vi "Analyze Coefficients-Quantized Multirate Filter.vi"() -> ()   [LabVIEW 2023]
doc: "Demonstrates how to use the DFD FXP MRate Quantization VI to quantize the coefficients of a floating-point multirate filter and use the DFD Plot MRate Freq Response VI to analyze a quantized multirate filter.\n\n1) Complete the following steps to use this VI.Run the VI. This VI designs a floating-point multirate filter with the specifications in the <B>Design Settings</B> section. This VI then quantize the multirate filter coefficients.\n2) Observe the Magnitude Responses graph. This graph displays the magnitude responses of both the fixed-point multirate filter and the reference floating-point multirate filter. You also can observe the Phase Responses graph for more information.\n3) Modify the <B>Quantization Settings</B> and run this VI again. Observe the Magnitude Responses graph to see how your changes affect the magnitude response of the fixed-point multirate filter.\n4) Examine the block diagram of this VI to obtain information about using the DFD FXP MRate Quantization Vi and the DFD Plot MRate Freq Response VI."
uses:
  <vilib>/addons/Digital Filter Design/_Objects.llb/DFD Multirate Filter Specification (Design).ctl
  <vilib>/addons/Digital Filter Design/_Objects.llb/DFD Filter Ripple Specification (Design).ctl
  <vilib>/addons/Digital Filter Design/_Objects.llb/DFD Coef Norm Type.ctl
  <vilib>/addons/Digital Filter Design/_Objects.llb/DFD Multirate Filtering Mode.ctl
  <vilib>/addons/Digital Filter Design/_Objects.llb/DFD Phase Setting.ctl
  <vilib>/addons/Digital Filter Design/Design.llb/DFD MRate Filter Design (Integer).vi
  <vilib>/addons/Digital Filter Design/NI_DigFilterLicensed.lvlib
panel:
  in  "dB on?":bool=TRUE
  in  "Phase View":T1
  out "Phase Responses":cluster{"f0":dbl, "df":dbl, "values":dbl[]}[](graph)
  out "Error Message":string
  out "Magnitude Responses":cluster{"f0":dbl, "df":dbl, "values":dbl[]}[](graph)
  in  "Filtering Mode":T2=2 items=["No Rate Change", "Interpolation", "Decimation"]
  in  "Factor":i32=8
  in  "Coefficients Word Length":i16=16
  in  "Scale by Power of 2?":bool
  in  "Scale Type":T3=enum."Time Domain 1-Norm"
  in  "Ripple Specifications":T4={"passband"=0.1, "stopband"=60.0, "dB/linear? (T: dB)"=TRUE}
  in  "Input Sampling Frequency [Hz]":dbl=800.0
  in  "Frequency Specifications [Hz]":T5={"fpass"=45.0, "fstop"=52.0}
  # "Select Help>>Show Context Help and move the cursor over the VI icon for more information."
  # "Design Settings"
  # "Quantization Settings"
  # "View Settings"
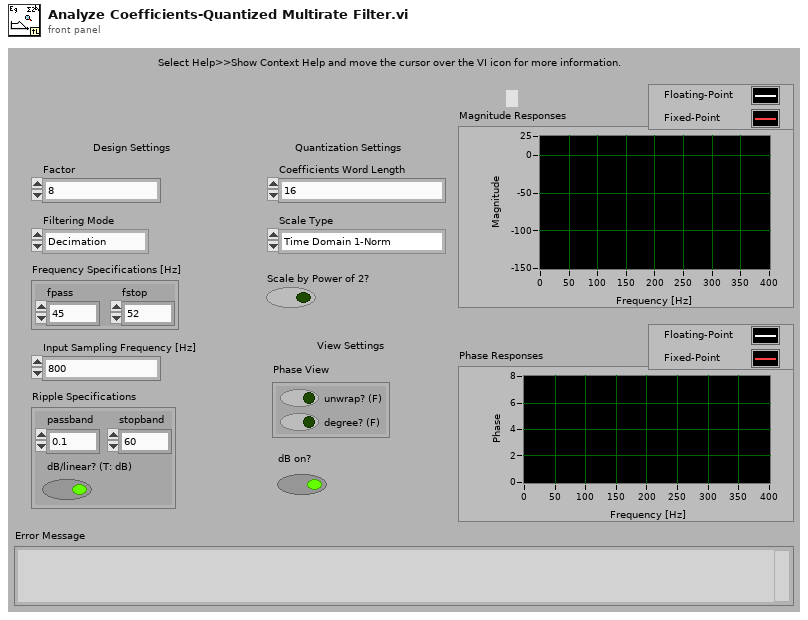
[diagram p1: front panel]
types:
  T1 = typedef "NI_DigFilterLicensed.lvlib/DFD Phase Setting.ctl" = cluster{"unwrap? (F)":bool, "degree? (F)":bool}
  T2 = typedef "NI_DigFilterLicensed.lvlib/DFD Multirate Filtering Mode.ctl" = u16
  T3 = typedef "NI_DigFilterLicensed.lvlib/DFD Coef Norm Type.ctl" = enum16{"No Norm", "Time Domain 1-Norm", "Time Domain 2-Norm", "Time Domain Inf-Norm"}
  T4 = typedef "NI_DigFilterLicensed.lvlib/DFD Filter Ripple Specification (Design).ctl" = cluster{"passband":dbl, "stopband":dbl, "dB/linear? (T: dB)":bool}
  T5 = typedef "NI_DigFilterLicensed.lvlib/DFD Multirate Filter Specification (Design).ctl" = cluster{"fpass":dbl, "fstop":dbl}
  T6 = typedef "NI_DigFilterLicensed.lvlib/DFD Multirate Filter Obj.ctl" = cluster{"mMRate_Structure":enum16{"CIC", "FIR", "IIR", "Lattice"}, "mMRate_Mode":T7, "mMRate_Factor":i32, "mMRate_FIRParams":cluster{"mMRate_FIR_H":dbl[], "mMRate_FIR_IsNyquist?":bool, "mMRate_FIR_IsSymmetric?":bool}, "mMRate_CICParams":cluster{"mMRate_CIC_#Stage":i32, "mMRate_CIC_Lag":i32, "mMRate_CIC_Type":enum16{"Lowpass", "Highpass"}}, "mMRate_Order":i32, "mMRate_Version":string, "mMRate_Comments":string, "mMRate_RationalFactor":cluster{"mMRate_L":i32, "mMRate_M":i32}, "mMRate_Fs":dbl, "mMRate_Quantized?":bool, "mMRate_QFilterGain":dbl, "mMRate_CoefWl":i16, "mMRate_Scaling":cluster{"mMRate_ScaleByPowerOf2?":bool, "mMRate_ScaleType":T3}, "mMRate_InputWl":i16, "mMRate_OutputWl":i16, "mMRate_OutputMode":T8, "mMRate_MultMode":T9, "mMRate_BitPruning":bool, "mMRate_GainWl":i16, "mMRate_OutputFwl":i16, "mMRate_SumIwl":i16, "mMRate_InputIwl ":i16, "mMRate_SumWl":i16, "mMRate_CoefIwl":i16}
  T7 = typedef "NI_DigFilterLicensed.lvlib/DFD Multirate Mode.ctl" = i16
  T8 = typedef "NI_DigFilterLicensed.lvlib/DFD Round-off Mode.ctl" = enum16{"Nearest", "Truncation"}
  T9 = typedef "NI_DigFilterLicensed.lvlib/DFD FXP MRate Multiply Mode.ctl" = enum16{"Truncated", "Full"}
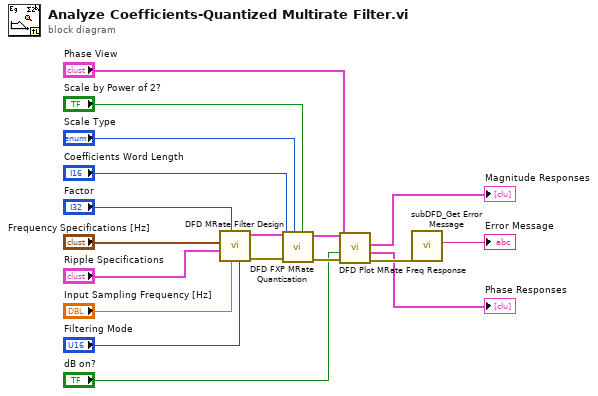
[diagram p0: block diagram]
diagram:
  n1 = call-poly <vilib>:"DFD MRate Filter Design.vi"("filtering mode"="Filtering Mode", "fs in [Hz]"="Input Sampling Frequency [Hz]", "factor"="Factor", "ripple specs"="Ripple Specifications", "freq specs [Hz]"="Frequency Specifications [Hz]") -> ("error out"=w17:errorcluster, "multirate filter out"=w18:T6)  [unwired: 3 in, 2 out]
  n2 = call <vilib>:"DFD FXP MRate Quantization.vi"("scale by power of 2? (F)"="Scale by Power of 2?", "scale type"="Scale Type", "error in (no error)"=w17, "coefficients word length"="Coefficients Word Length", "multirate filter in"=w18) -> ("error out"=w8:errorcluster, "multirate filter out"=w9:T6)  [unwired: 1 in, 4 out]
  n3 = call <vilib>:"DFD Plot MRate Freq Response.vi"("error in (no error)"=w8, "dB on? (T)"="dB on?", "phase view"="Phase View", "multirate filter in"=w9) -> ("error out"=w5:errorcluster, "phase response"=→"Phase Responses":cluster{"f0":dbl, "df":dbl, "values":dbl[]}[], "magnitude response"=→"Magnitude Responses":cluster{"f0":dbl, "df":dbl, "values":dbl[]}[])  [unwired: 3 in, 2 out]
  n4 = call <vilib>:"subDFD_Get Error Message.vi"("error in (no error)"=w5) -> ("Error Message"=→"Error Message":string)  [unwired: 10 out]
